vi "mergePrograms.vi"(7 "init":bool, 9 "syncLabel":u8, 10 "sceneReplaceList":i32[][](array[numeric]), 11 "editArray":T1[](array[typedef])) -> (3 "editRecalc":T1[](array[typedef]))   [LabVIEW 2014]
uses:
  typeDefs/editControl.ctl
  typeDefs/variantFlat.ctl
  typeDefs/poiCommand.ctl
  typeDefs/sceneControlType.ctl
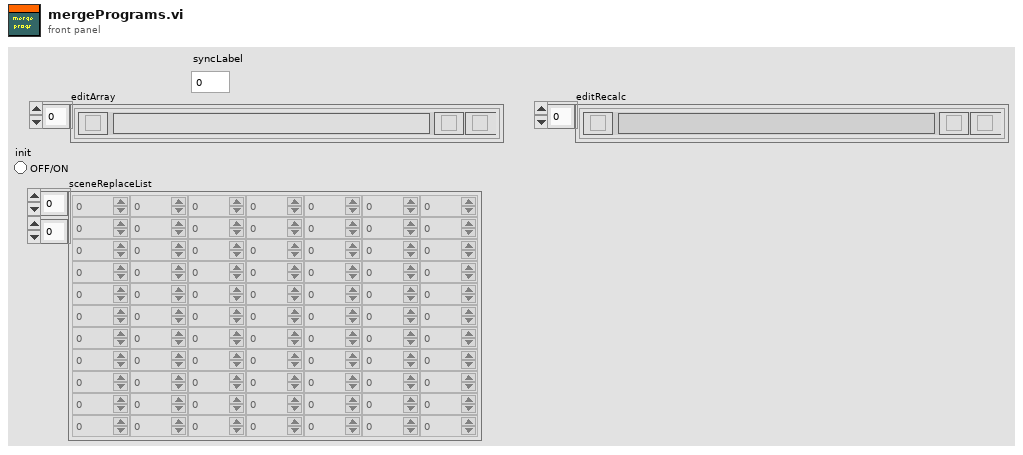
[diagram p1: front panel]
types:
  T1 = typedef "editControl.ctl" = cluster{"edit":bool, "info":string, "variantFlat":T2, "codeCluster":cluster{"code":u8[][]}, "del":bool, "ins":bool}
  T2 = typedef "variantFlat.ctl" = cluster{"type string":i16[], "data string":string}
  T3 = typedef "poiCommand.ctl" = u8
  T4 = typedef "sceneControlType.ctl" = enum16{"Ende", "label", "syncPoint", "play", "loop", "setActiveScene", "presetRGB", "fadeToRGB", "fadeToFrame", "jumpTo", "dimm", "allOneColor"}
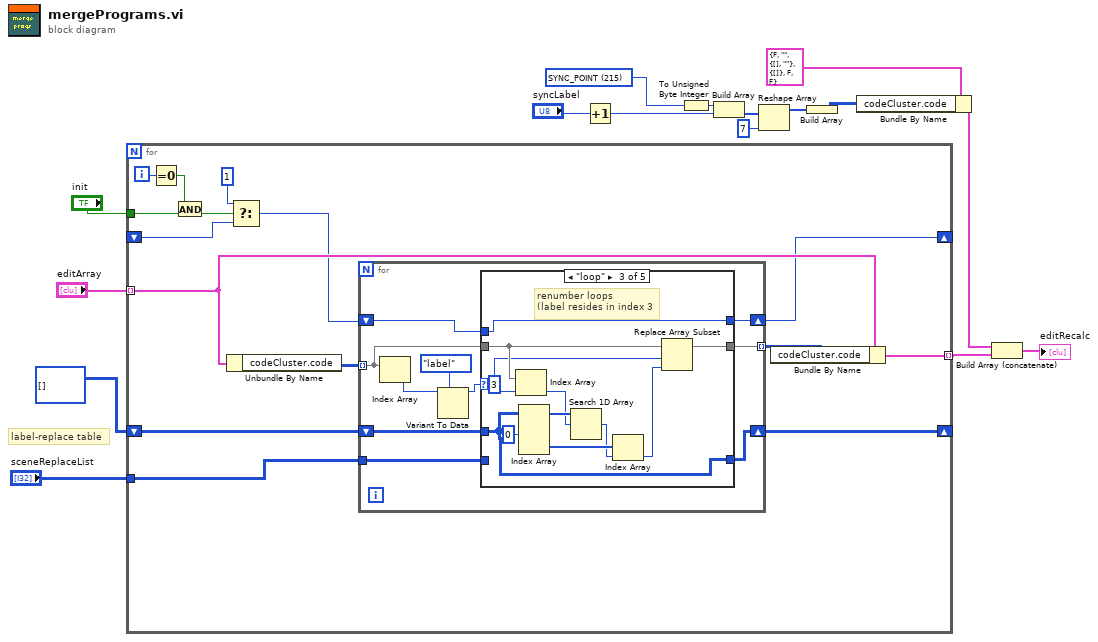
[diagram p0: block diagram]
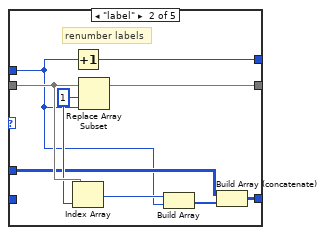
[diagram p3: hidden frame]
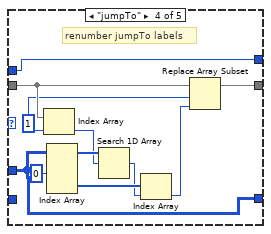
[diagram p4: hidden frame]
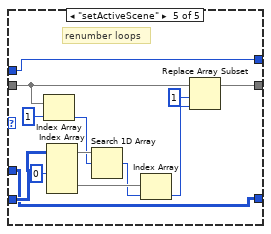
[diagram p5: hidden frame]
diagram:
  w1 = T3 215 items=["SET_PIXEL"=0, "HEAD_SCENE"=192, "TAIL_SCENE"=193, "SAVE_SCENE"=194, "HEAD_PROG"=195, "TAIL_PROG"=196, "SAVE_PROG"=197, "INIT_FLASH"=198, "LOAD_SCENE"=199, "SHOW_RGB"=200, "PLAY_FRAMES"=201, "ANIMATE"=202, "DISPLAY_IP"=203, "DIMM"=204, "FADE2FRAME"=205, "START_PROG"=206, "STOP_PROC"=207, "PAUSE_PROC"=208, "JUMP2SYNC"=209, "CONNECT"=210, "DISCONNECT"=211, "CLIENT_DISCON"=212, "USE_SSID"=213, "LOOP_START"=214, "SYNC_POINT"=215, "LOOP_END"=216] ("Ring")
  # "label-replace table"
  n1 = for {
    tunnel: "editArray" -> [w31] mode=indexing
    tunnel: [w30] -> w16 mode=indexing
    shift-right: [w28] -> _
    shift-left: _ -> [w24]
    tunnel: "init" -> [w25]
    shift-right: [w20] -> _
    shift-left: i32[][] [] ("t") -> [w17]
    tunnel: "sceneReplaceList" -> [w18]
    i -> [w22]
    n2 = Equal To 0?(x=w22) -> (x = 0?=w21:bool)
    n3 = And(x=w21, y=w25) -> (x .and. y?=w19:bool)
    n4 = Unbundle By Name(w31) -> ("codeCluster.code"=w29:u8[][])
    n5 = Select(t=1, s=w19, f=w24) -> (s? t:f=w23:i32)
    n6 = for {
      tunnel: w29 -> [w41] mode=indexing
      shift-right: [w39] -> w28
      shift-left: w23 -> [w40]
      tunnel: [w38] -> w27 mode=indexing
      shift-right: [w36] -> w20
      shift-left: w17 -> [w37]
      tunnel: w18 -> [w32]
      n7 = Index Array(array=w41) -> (element=w35:u8)  [unwired: 1 in]
      n8 = Variant To Data(type=sceneControlType."label" ("prog"), Variant=w35) -> (data=w33:T4)  [unwired: 1 in, 1 out]
      n9 = case shown="\"loop\"" w33 {
        tunnel: w41 -> [w43 w51 w63 w74 w86]
        tunnel: w40 -> [w44 w45 w62 w73 w85]
        tunnel: [w44 w53 w62 w73 w85] -> w39
        tunnel: [w43 w52 w64 w75 w88] -> w38
        tunnel: w37 -> [w42 w48 w58 w69 w76]
        tunnel: [w42 w47 w58 w69 w76] -> w36
        tunnel: w32 -> [_ _ _ _ w77]
        frame "Ende", Default {
        }
        frame "label" {
          w50 = 1 ("index")
          # "renumber labels"
          n10 = Increment(x=w45) -> (x+1=w53:i32)
          n11 = Index Array(array=w51, index=w50) -> (element=w46:u8)
          n12 = Replace Array Subset(array=w51, new element=w45, index=w50) -> (w52:u8[])
          n13 = Build Array(w46, w45) -> (w49:i32[])
          n14 = Build Array (concatenate)(w48, w49) -> (w47:i32[][])
        }
        frame "loop" {
          w54 = 3 ("index")
          # "renumber loops\n(label resides in index 3"
          n15 = Index Array(array=w63, index=w54) -> (element=w60:u8)
          n16 = Index Array(array=w58, index (col) #1=0 ("disabled index (col)")) -> (element #1=w61:i32[], element #2=w57:i32[])  [unwired: 3 in]
          n17 = Search 1D Array(1D array=w61, element=w60) -> (index of element=w56:i32)  [unwired: 1 in]
          n18 = Index Array(array=w57, index=w56) -> (element=w55:i32)
          n19 = Replace Array Subset(array=w63, new element=w55, index=w54) -> (w64:u8[])
        }
        frame "jumpTo" {
          w65 = 1 ("index")
          # "renumber jumpTo labels"
          n20 = Index Array(array=w74, index=w65) -> (element=w71:u8)
          n21 = Index Array(array=w69, index (col) #1=0 ("disabled index (col)")) -> (element #1=w72:i32[], element #2=w68:i32[])  [unwired: 3 in]
          n22 = Search 1D Array(1D array=w72, element=w71) -> (index of element=w67:i32)  [unwired: 1 in]
          n23 = Index Array(array=w68, index=w67) -> (element=w66:i32)
          n24 = Replace Array Subset(array=w74, new element=w66, index=w65) -> (w75:u8[])
        }
        frame "setActiveScene" {
          # "renumber loops"
          n25 = Index Array(array=w86, index=1) -> (element=w82:u8)
          n26 = Index Array(array=w77, index (col) #1=0 ("disabled index (col)")) -> (element #1=w83:i32[], element #2=w80:i32[])  [unwired: 3 in]
          n27 = Search 1D Array(1D array=w83, element=w82) -> (index of element=w79:i32)  [unwired: 1 in]
          n28 = Index Array(array=w80, index=w79) -> (element=w78:i32)
          n29 = Replace Array Subset(array=w86, new element=w78, index=1) -> (w88:u8[])
        }
      }
    }
    n30 = Bundle By Name(cluster=w31, "codeCluster.code"=w27) -> (w30:T1)
  }
  n31 = Increment(x="syncLabel") -> (x+1=w2:u8)
  n32 = To Unsigned Byte Integer(number=w1) -> (unsigned 8bit integer=w8:T3)
  n33 = Build Array(w8, w2) -> (w7:T3[])
  n34 = Reshape Array(w7, 7 ("dimension size")) -> (w5:T3[])
  n35 = Build Array(w5) -> (w4:T3[][])
  n36 = Bundle By Name(cluster=T1 {"edit"=FALSE, "info"="", "variantFlat"={"type string"=[], "data string"=""}, "codeCluster"={"code"=[]}, "del"=FALSE, "ins"=FALSE} ("editCntrl"), "codeCluster.code"=w4) -> (w3:T1)
  n37 = Build Array (concatenate)(w3, w16) -> (→"editRecalc":T1[])
